vi "Tree_Select first item.vi"(11 "Tree ref":refnum<vi>) -> ()   [LabVIEW 2023]
doc: "Select first item in tree that is not disabled after making the tree key focus."
panel:
  in  "Tree":string[](tree)
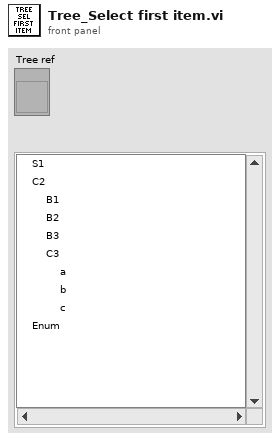
[diagram p1: front panel]
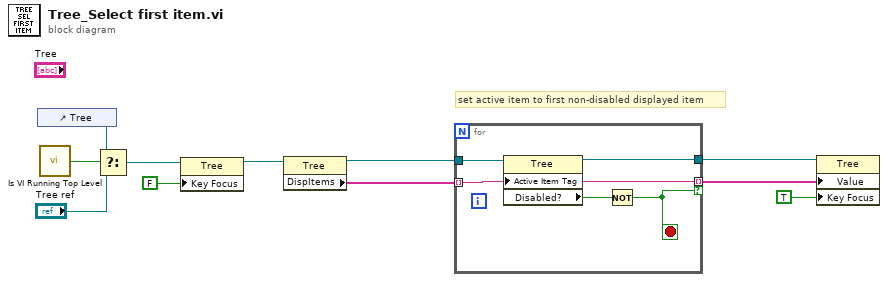
[diagram p0: block diagram]
diagram:
  # "set active item to first non-disabled displayed item"
  n1 = control-ref of="Tree"() -> (w10:refnum<vi>)
  n2 = call "Is VI Running Top Level.vi"() -> ("Top Level?"=w11:bool)  [unwired: 5 in]
  n3 = Select(t=w10, s=w11, f="Tree ref") -> (s? t:f=w8:refnum<vi>)
  n4 = property class="Tree"(reference=w8, "Key Focus"=FALSE) -> (reference out=w3:refnum<vi>)  [unwired: 1 in, 1 out]
  n5 = property class="Tree"(reference=w3) -> (reference out=w7:refnum<vi>, "DispItems"=w6:string[])  [unwired: 1 in, 1 out]
  n6 = for {
    tunnel: w7 -> [w16]
    tunnel: w6 -> [w13] mode=indexing
    tunnel: [w14] -> w5
    tunnel: [w13] -> w2 mode=indexing if=w12
    stop <- w12 stop-if-true
    n7 = property class="Tree"(reference=w16, "Active Item Tag"=w13) -> (reference out=w14:refnum<vi>, "Disabled?"=w15:bool)  [unwired: 1 in, 1 out]
    n8 = Not(x=w15) -> (.not. x?=w12:bool)
  }
  n9 = property class="Tree"(reference=w5, "Value"=w2, "Key Focus"=TRUE) -> ()  [unwired: 1 in, 2 out]
